vi "Redraw AOIs.vi"(0 "Resize to Image Size?":bool, 3 "Image Src (Red Plane)":T1, 4 "Window Number (0...15)":i32, 5 "Image Src (RGB)":T1) -> (2 "Image Dst Out (RGB)":T1)   [LabVIEW 2011]
doc: "Redraws AOIs listed in the global multiple AOI list into the red pane, then adds this to the red pane to the RGB image and displays it."
uses:
  <vilib>/vision/Image Controls.llb/IMAQ Image.ctl
  AOI List Globals.vi
  <vilib>/vision/NI_Vision_Development_Module.lvlib
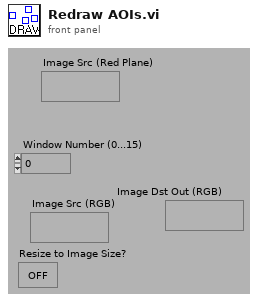
[diagram p1: front panel]
types:
  T1 = typedef "IMAQ Image.ctl" = refnum<image>
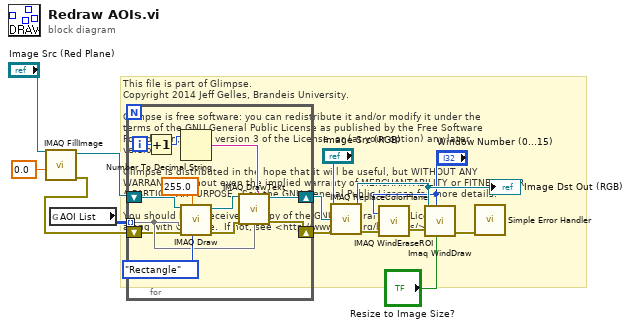
[diagram p0: block diagram]
diagram:
  # "This file is part of Glimpse. \nCopyright 2014 Jeff Gelles, Brandeis University.    \n\nGlimpse is free software: you can redistribute it and/or modify it under the \nterms of the GNU General Public License as published by the Free Software \nFoundation, either version 3 of the License, or (at your option) any later \nversion.\n\nGlimpse is distributed in the hope that it will be useful, but WITHOUT ANY \nWARRANTY; without even the implied warranty of MERCHANTABILITY or FITNESS FOR \nA PARTICULAR PURPOSE.  See the GNU General Public License for more details.\n\nYou should have received a copy of the GNU General Public License\nalong with Glimpse.  If not, see <http://www.gnu.org/licenses/>."
  n1 = call "IMAQ FillImage"("Pixel Value (U8, U16, I16, Float)"=sgl 0.0 ("Pixel Value (U8, I16, Float)"), "Image"="Image Src (Red Plane)") -> ("error out"=w7:errorcluster, "Image Out"=w8:T1)  [unwired: 5 in, 3 out]
  n2 = global read "AOI List Globals.vi" "AOI List"() -> (w11:u16[][])
  n3 = for {
    tunnel: w11 -> [w20] mode=indexing
    shift-right: [w17] -> w10
    shift-left: w7 -> [w19]
    shift-right: [w23] -> w2
    shift-left: w8 -> [w25]
    i -> [w22]
    n4 = Increment(x=w22) -> (x+1=w15:i32)
    n5 = Number To Decimal String(number=w15) -> (decimal integer string=w21:string)  [unwired: 1 out]
    n6 = call "IMAQ Draw"("Shape to draw"=enum32{"Line", "Rectangle", "Oval"}."Rectangle", "Pixel Color"=sgl 255.0, "error in (no error)"=w19, "Coordinates"=w20, "Image Src"=w25) -> ("error out"=w18:errorcluster, "Image Dst Out"=w16:T1)  [unwired: 2 in, 3 out]
    n7 = call "IMAQ DrawText"("String"=w21, "Insertion Point"=w20, "error in (no error)"=w18, "Image Src"=w16) -> ("error out"=w17:errorcluster, "Image Dst Out"=w23:T1)  [unwired: 3 in, 3 out]
  }
  n8 = call "IMAQ ReplaceColorPlane"("Image Src"="Image Src (RGB)", "Red or Hue Plane"=w2, "error in (no error)"=w10) -> ("Image Dst Out"=w13:T1, "error out"=w3:errorcluster)  [unwired: 4 in, 7 out]
  "Image Dst Out (RGB)" <- w13
  n9 = call "IMAQ WindEraseROI"("Window Number"="Window Number (0...15)", "error in (no error)"=w3) -> ("error out"=w4:errorcluster)  [unwired: 4 out]
  n10 = call "Imaq WindDraw"("Resize to Image Size? (Y)"="Resize to Image Size?", "Window Number (0...15)"="Window Number (0...15)", "error in (no error)"=w4, "Image"=w13) -> ("error out"=w12:errorcluster)  [unwired: 2 in, 5 out]
  n11 = call <vilib>:"Simple Error Handler.vi"("error in (no error)"=w12) -> ()  [unwired: 1 in, 8 out]
